vi "Get Class Name.vi"(1 "Basic DAQ Board in":refnum<class "Basic DAQ Design.lvclass">) -> (0 "class name":string)   [LabVIEW 2023, in "Basic DAQ Design.lvclass"]
doc: "Get the name of this class."
uses:
  Basic DAQ Design.lvclass
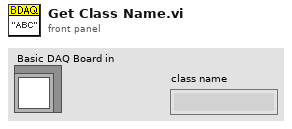
[diagram p1: front panel]
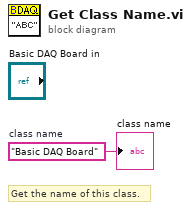
[diagram p0: block diagram]
diagram:
  w1 = "Basic DAQ Board"  # class name
  # "Get the name of this class."
  "class name" <- w1
